vi "program.vi"() -> (0 "Vaporizer Status":bool, 4 "Cooler Status":bool, 5 "Filter Status":bool, 6 "Recovery Filter Status":bool, 7 "Compressor Status":bool, 9 "Mixer Status":bool, 10 "Condensor Status":bool, 11 "Converter Status":bool, 13 "Ammonia Flow Rate":dbl(knob) scale=0.0..10.0, 15 "Absorption Tank  Status":bool)   [LabVIEW 2021]
uses:
  5dba2dd3-3eb6-47e8-980b-4a7fe52b60dd.vi
  aa427e9b-4a00-4a3c-8f1e-02a1676d43b3.vi
  c319c837-4be1-48ba-bc3d-b9c54b653514.vi
  a9099b65-414a-4ebe-9c07-2ab086c03dab.vi
  1b0875cc-9c07-4af8-a27b-c6ad72a29e72.vi
  cfb05d54-3552-4b18-86e4-2782e9494e5d.vi
  <vilib>/express/express arith-compare/Formula/XNode/ExpressFormulaBlockNode.xnode
panel:
  out "Current Production Cost":dbl
  out "Price of Liquid Ammonia":dbl
  in  "stop":bool
  in  "Path":path
  in  "Valve 2":bool
  out "Litres":dbl
  out "Liters Dispensed":dbl
  out "Liters Dispensed 2":dbl
  in  "Valve":bool
  in  "Run Plant":bool
  out "Filter":bool
  in  "Cooling Temp 1":dbl(slide) scale=100.0..200.0
  in  "Cooling Temp 2":dbl(slide) scale=10.0..100.0
  in  "Converter Pressure":dbl(slide) scale=0.0..4.0
  in  "Water Flow Rate Slide":dbl(slide) scale=0.0..10.0
  in  "Tower Pressure":dbl(slide) scale=7.0..14.0
  in  "Tower Temperature":dbl(slide) scale=0.0..100.0
  in  "Converter Temperature":dbl(slide) scale=500.0..1200.0
  out "Tower Pressure":dbl(knob) scale=7.0..14.0
  out "Converter Pressure":dbl(knob) scale=0.0..4.0
  out "Water Flow Rate":dbl(knob) scale=0.0..10.0
  out "Storage Tank":dbl(slide) scale=0.0..1000.0
  out "Absorption Tower":bool
  out "Condensor":bool
  out "Catayltic Recovery Filter":bool
  out "Cooler":bool
  out "Converter":bool
  in  "Air flow rate set":dbl(slide) scale=0.0..10.0
  out "Mixer":bool
  out "Air Flow Rate":dbl(knob) scale=0.0..10.0
  out "Compressor":bool
  in  "Ammonia Flow Rate":dbl(slide) scale=0.0..10.0
  out "Vaporizer":bool
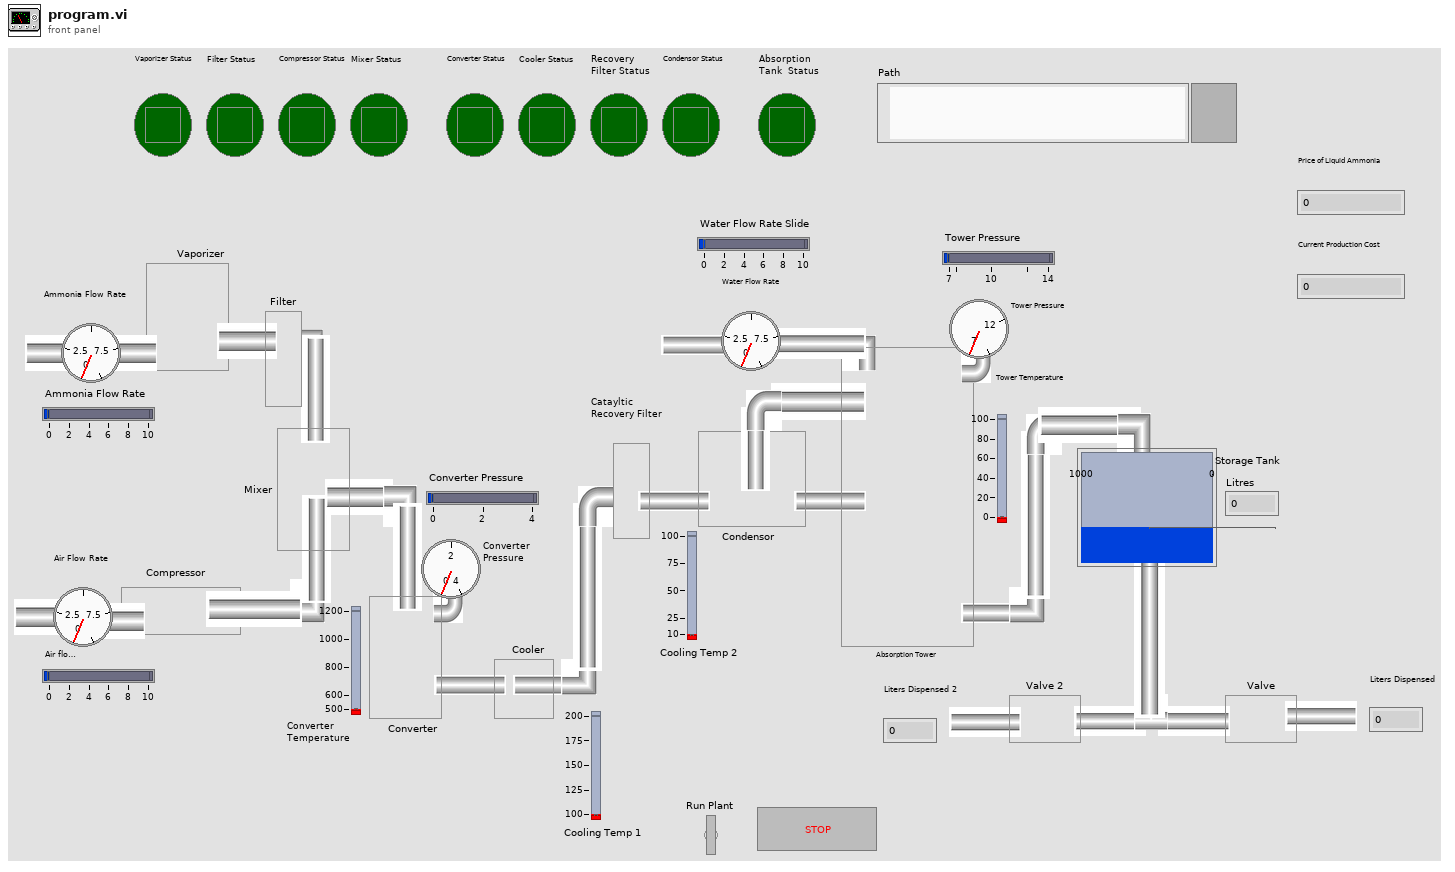
[diagram p1: front panel]
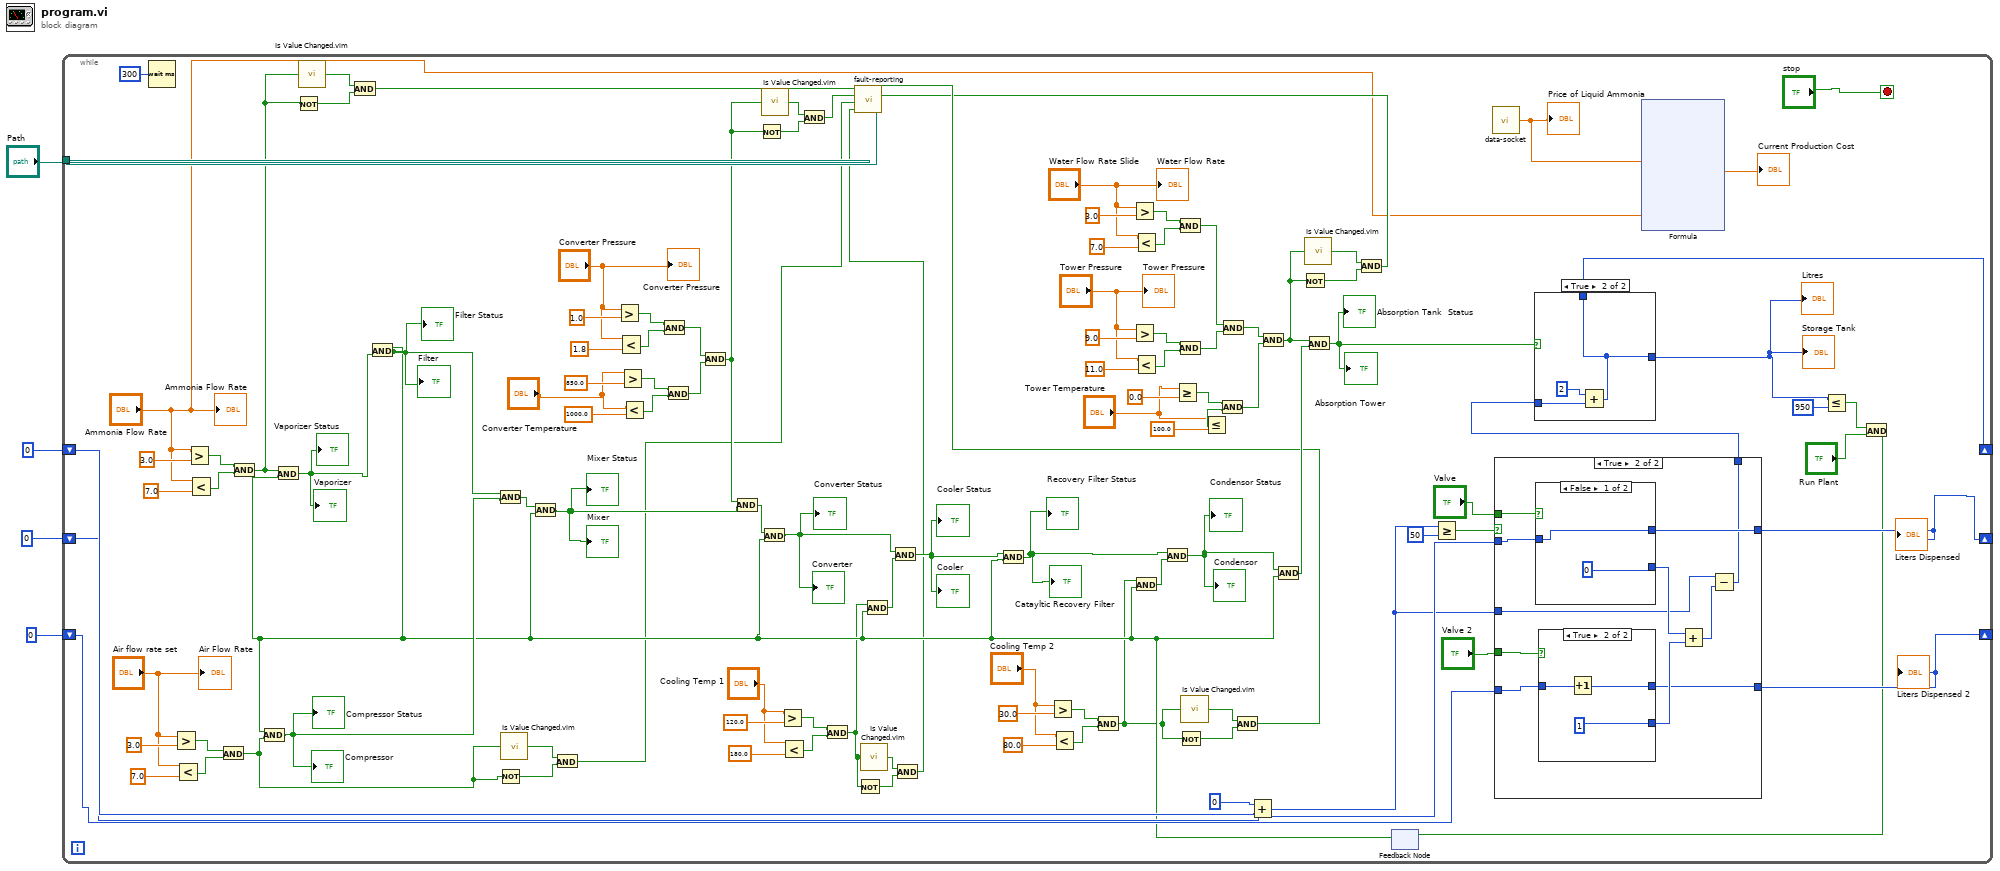
[diagram p0: block diagram]
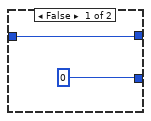
[diagram p3: hidden frame]
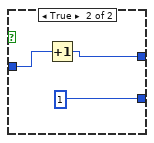
[diagram p4: hidden frame]
diagram:
  n1 = while {
    shift-right: [w50] -> _
    shift-left: 0 -> [w52]
    shift-right: [w46] -> _
    shift-left: 0 -> [w47]
    shift-right: [w42] -> _
    shift-left: 0 -> [w44]
    tunnel: "Path" -> [w32]
    stop <- "stop" stop-if-true
    n2 = Wait (ms)(milliseconds to wait=u32 300) -> ()  [unwired: 1 out]
    n3 = Greater?(x="Air flow rate set", y=3.0) -> (0:w73:bool)
    n4 = Less?(x="Air flow rate set", y=7.0) -> (x < y?=w72:bool)
    n5 = Greater?(x="Ammonia Flow Rate", y=3.0) -> (0:w77:bool)
    n6 = Less?(x="Ammonia Flow Rate", y=7.0) -> (x < y?=w76:bool)
    n7 = And(x=w73, y=w72) -> (x .and. y?=w21:bool)
    n8 = And(x=w77, y=w76) -> (x .and. y?=w31:bool)
    n9 = Not(x=w31) -> (.not. x?=w29:bool)
    n10 = call "Is Value Changed.vim"("value"=w31) -> ("changed or first call?"=w30:bool)
    n11 = And(x=w30, y=w29) -> (x .and. y?=w28:bool)
    n12 = Not(x=w21) -> (.not. x?=w22:bool)
    n13 = call "Is Value Changed.vim"("value"=w21) -> ("changed or first call?"=w23:bool)
    n14 = And(x=w23, y=w22) -> (x .and. y?=w20:bool)
    n15 = Greater?(x="Converter Pressure", y=1.0) -> (0:w110:bool)
    n16 = Less?(x="Converter Pressure", y=1.8) -> (x < y?=w109:bool)
    n17 = Greater?(x="Converter Temperature", y=850.0) -> (0:w106:bool)
    n18 = Less?(x="Converter Temperature", y=1000.0) -> (x < y?=w105:bool)
    n19 = And(x=w110, y=w109) -> (x .and. y?=w103:bool)
    n20 = And(x=w106, y=w105) -> (x .and. y?=w102:bool)
    n21 = And(x=w103, y=w102) -> (x .and. y?=w25:bool)
    n22 = Not(x=w25) -> (.not. x?=w26:bool)
    n23 = call "Is Value Changed.vim"("value"=w25) -> ("changed or first call?"=w27:bool)
    n24 = Greater?(x="Cooling Temp 1", y=120.0) -> (0:w97:bool)
    n25 = Less?(x="Cooling Temp 1", y=180.0) -> (x < y?=w96:bool)
    n26 = And(x=w27, y=w26) -> (x .and. y?=w24:bool)
    n27 = And(x=w97, y=w96) -> (x .and. y?=w17:bool)
    n28 = Not(x=w17) -> (.not. x?=w18:bool)
    n29 = call "Is Value Changed.vim"("value"=w17) -> ("changed or first call?"=w19:bool)
    n30 = And(x=w19, y=w18) -> (x .and. y?=w16:bool)
    n31 = Greater?(x="Cooling Temp 2", y=30.0) -> (0:w91:bool)
    n32 = Less?(x="Cooling Temp 2", y=80.0) -> (x < y?=w90:bool)
    n33 = And(x=w91, y=w90) -> (x .and. y?=w13:bool)
    n34 = Greater?(x="Water Flow Rate Slide", y=3.0) -> (0:w82:bool)
    n35 = Greater?(x="Tower Pressure", y=9.0) -> (0:w68:bool)
    n36 = Less?(x="Water Flow Rate Slide", y=7.0) -> (x < y?=w81:bool)
    n37 = Less?(x="Tower Pressure", y=11.0) -> (x < y?=w67:bool)
    n38 = Greater Or Equal?(x="Tower Temperature", y=0.0) -> (x >= y?=w63:bool)
    n39 = And(x=w82, y=w81) -> (x .and. y?=w60:bool)
    n40 = And(x=w68, y=w67) -> (x .and. y?=w59:bool)
    n41 = Not(x=w13) -> (.not. x?=w14:bool)
    n42 = call "Is Value Changed.vim"("value"=w13) -> ("changed or first call?"=w15:bool)
    n43 = Less Or Equal?(x="Tower Temperature", y=100.0) -> (x <= y?=w62:bool)
    n44 = And(x=w63, y=w62) -> (x .and. y?=w57:bool)
    n45 = And(x=w60, y=w59) -> (x .and. y?=w58:bool)
    n46 = And(x=w15, y=w14) -> (x .and. y?=w12:bool)
    n47 = Add(x=0, y=w52) -> (x+y=w41:i32)
    n48 = And(x=w58, y=w57) -> (x .and. y?=w9:bool)
    n49 = Not(x=w9) -> (.not. x?=w10:bool)
    n50 = call "Is Value Changed.vim"("value"=w9) -> ("changed or first call?"=w11:bool)
    n51 = And(x=w11, y=w10) -> (x .and. y?=w8:bool)
    n52 = call "fault-reporting.vi"("Path"=w32, "Tower"=w8, "Condensor"=w12, "Cooler"=w16, "Air"=w20, "Converter"=w24, "Ammonia"=w28) -> ()  [unwired: 1 in]
    n53 = feedback #1() -> (w34:bool)  [unwired: 1 in]
    n54 = And(x=w34, y=w21) -> (x .and. y?=w114:bool)
    "Compressor" <- w114
    "Compressor Status" <- w114
    n55 = And(x=w31, y=w34) -> (x .and. y?=w117:bool)
    "Vaporizer" <- w117
    "Vaporizer Status" <- w117
    n56 = And(x=w34, y=w117) -> (x .and. y?=w115:bool)
    "Filter" <- w115
    "Filter Status" <- w115
    n57 = And(x=w115, y=w114) -> (x .and. y?=w116:bool)
    n58 = And(x=w116, y=w34) -> (x .and. y?=w101:bool)
    "Mixer" <- w101
    "Mixer Status" <- w101
    n59 = And(x=w25, y=w101) -> (x .and. y?=w100:bool)
    n60 = And(x=w100, y=w34) -> (x .and. y?=w94:bool)
    "Converter" <- w94
    "Converter Status" <- w94
    n61 = And(x=w17, y=w34) -> (x .and. y?=w89:bool)
    n62 = And(x=w94, y=w89) -> (x .and. y?=w88:bool)
    "Cooler" <- w88
    "Cooler Status" <- w88
    n63 = And(x=w88, y=w34) -> (x .and. y?=w86:bool)
    "Catayltic Recovery Filter" <- w86
    "Recovery Filter Status" <- w86
    n64 = And(x=w13, y=w34) -> (x .and. y?=w87:bool)
    n65 = And(x=w86, y=w87) -> (x .and. y?=w56:bool)
    "Condensor" <- w56
    "Condensor Status" <- w56
    n66 = And(x=w56, y=w34) -> (x .and. y?=w55:bool)
    n67 = And(x=w9, y=w55) -> (x .and. y?=w54:bool)
    "Absorption Tower" <- w54
    "Absorption Tank  Status" <- w54
    n68 = Greater Or Equal?(x=w41, y=50) -> (x >= y?=w48:bool)
    n69 = call "data-socket.vi"() -> ("Price of Liquid Ammonia"=w7:dbl)  [unwired: 2 in]
    "Price of Liquid Ammonia" <- w7
    n70 = case shown="True" w48 {
      tunnel: w47 -> [w130 w141]
      tunnel: [w130 w140] -> w46
      tunnel: "Valve" -> [_ w139]
      tunnel: w44 -> [w129 w138]
      tunnel: "Valve 2" -> [_ w137]
      tunnel: [w129 w131] -> w42
      tunnel: w41 -> [w128 w133]
      tunnel: [w128 w132] -> w40
      frame False {
      }
      frame True {
        n71 = case shown="False" w139 {
          tunnel: w141 -> [w148 w151]
          tunnel: [w148 w150] -> w140
          tunnel: [0 1] -> w136
          frame False {
          }
          frame True {
            n72 = Increment(x=w151) -> (x+1=w150:i32)
          }
        }
        n73 = case shown="True" w137 {
          tunnel: w138 -> [w143 w146]
          tunnel: [w143 w145] -> w131
          tunnel: [0 1] -> w135
          frame False {
          }
          frame True {
            n74 = Increment(x=w146) -> (x+1=w145:i32)
          }
        }
        n75 = Add(x=w136, y=w135) -> (x+y=w134:i32)
        n76 = Subtract(x=w133, y=w134) -> (x-y=w132:i32)
      }
    }
    "Liters Dispensed" <- w46
    "Liters Dispensed 2" <- w42
    n77 = case shown="True" w54 {
      tunnel: w40 -> [w152 w155]
      tunnel: [w152 w154] -> w50
      tunnel: [w152 w154] -> w39
      frame False {
      }
      frame True {
        n78 = Add(x=2, y=w155) -> (x+y=w154:i32)
      }
    }
    "Storage Tank" <- w39
    "Litres" <- w39
    n79 = xnode "Formula"("X1"=w7, "X2"="Ammonia Flow Rate") -> ("Result"=→"Current Production Cost":dbl)  [unwired: 1 in, 1 out]
    n80 = Less Or Equal?(x=w39, y=950) -> (x <= y?=w36:bool)
    n81 = And(x=w36, y="Run Plant") -> (x .and. y?=w35:bool)
    n82 = feedback-in #1(w35) -> ()
    "Ammonia Flow Rate" <- "Ammonia Flow Rate"
    "Air Flow Rate" <- "Air flow rate set"
    "Water Flow Rate" <- "Water Flow Rate Slide"
    "Converter Pressure" <- "Converter Pressure"
    "Tower Pressure" <- "Tower Pressure"
  }
